vi "initialize.vi"(0 "HGF_DSCEvent":refnum<class "HGF_DSCEvent.lvclass">, 3 "initializationData":variant, 5 "error in (no error)":errorcluster, 7 "binaryString":string, 8 "I8 Array":i8[](array[numeric]), 9 "prependSize? (T)":bool, 11 "byteOrder (0:big-endian, network order)":T1(ring)) -> (14 "dup HGF_DSCEvent":refnum<class "HGF_DSCEvent.lvclass">, 17 "found?":bool, 19 "error out":errorcluster)   [LabVIEW 2012, in "HGF_DSC.lvlib" / "HGF_DSCEvent.lvclass"]
doc: "This is a dynamic dispatch VI to be implemented by child classes to initialize their attributes.\n\n<B>Recommendation:</B> Use Variant for initialization data."
uses:
  HGF_DSCEvent.lvclass
  HGF_BaseClasses/HGF_NetworkVisitor/HGF_NetworkVisitor.lvclass
  HGF_BaseClasses/HGF_Event/HGF_Event.lvclass
  HGF_SV/HGF_SVEvent/HGF_SVEvent.lvclass
  HGF_DSCEvent.lvclass/HGF_DSCEvent.ctl
  HGF_DSCCommand/HGF_DSCCommand.lvclass
  HGF_DSCFactory/HGF_DSCFactory.lvclass
  HGF_DSCSubscriber/HGF_DSCSubscriber.lvclass
  HGF_BaseClasses/HGF_NetworkEvent/HGF_NetworkEvent.lvclass/HGF_NetworkEvent.lvclass
  HGF_BaseClasses/HGF_Factory/HGF_Factory.lvclass
  HGF_SV/Visitors/HGF_SVMonitorVisitor_register/HGF_SVMonitorVisitor_register.lvclass
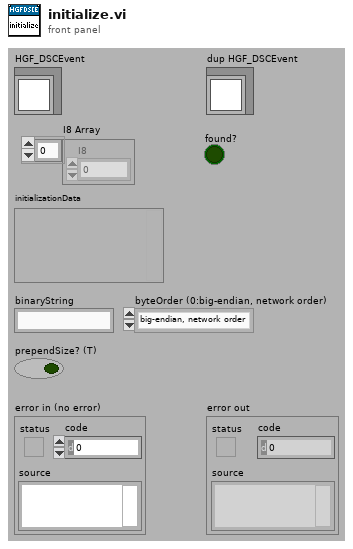
[diagram p1: front panel]
types:
  T1 = enum16{"big-endian, network order", "native, host order", "little-endian"}
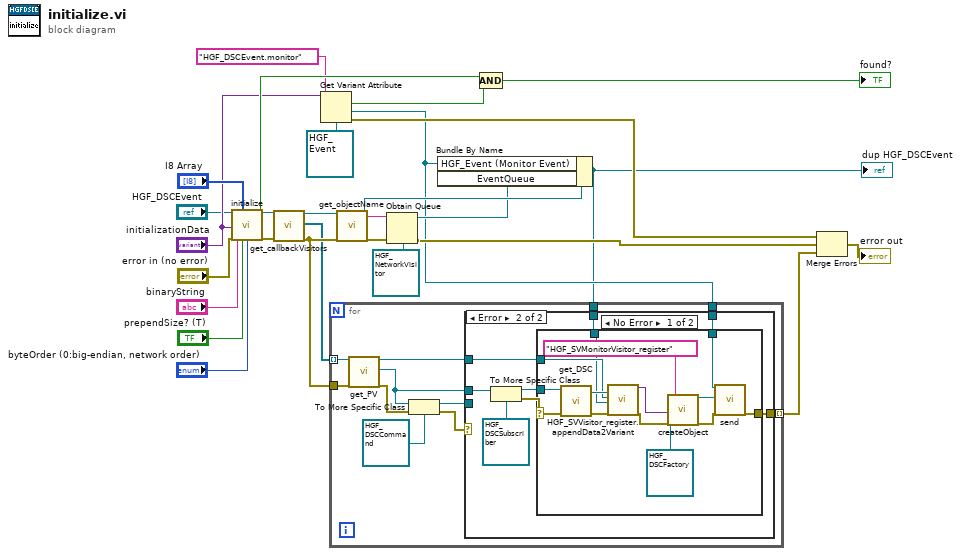
[diagram p0: block diagram]
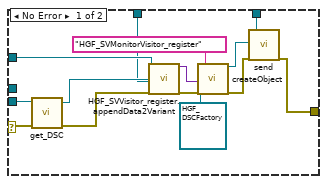
[diagram p2: hidden frame]
diagram:
  n1 = call-parent "initialize.vi"("HGF_SVEvent"="HGF_DSCEvent", "initializationData"="initializationData", "error in (no error)"="error in (no error)", "binaryString"="binaryString", "I8 Array"="I8 Array", "prependSize? (T)"="prependSize? (T)", "byteOrder (0:big-endian, network order)"="byteOrder (0:big-endian, network order)") -> ("dup HGF_SVEvent"=w6:refnum<class "HGF_DSCEvent.lvclass">, "found?"=w22:bool, "error out"=w4:errorcluster)  [unwired: 10 out]
  n2 = call "get_callbackVisitors.vi"("HGF_NetworkEvent"=w6, "error in (no error)"=w4) -> ("dup HGF_NetworkEvent"=w17:refnum<class "HGF_DSCEvent.lvclass">, "callbackVisitors"=w27:refnum<class "HGF_NetworkVisitor.lvclass">[], "error out"=w28:errorcluster)  [unwired: 15 out]
  n3 = Get Variant Attribute(Variant="initializationData", name="HGF_DSCEvent.monitor", default value (empty Variant)=refnum<class "HGF_Event.lvclass"> refnum ("HGF_BaseClasses.lvlib:HGF_Event.lvclass")) -> (found=w9:bool, value=w2:refnum<class "HGF_Event.lvclass">, error out=w5:errorcluster)  [unwired: 1 in, 1 out]
  n4 = call "get_objectName.vi"("HGF_Factory"=w17, "error in (no error)"=w28) -> ("dup HGF_Factory"=w16:refnum<class "HGF_DSCEvent.lvclass">, "objectName"=w13:string, "error out"=w15:errorcluster)  [unwired: 15 out]
  n5 = Obtain Queue(name (unnamed)=w13, element data type=refnum<class "HGF_NetworkVisitor.lvclass"> refnum ("HGF_BaseClasses.lvlib:HGF_NetworkVisitor.lvclass"), error in (no error)=w15) -> (queue out=w8:refnum<queue>, error out=w14:errorcluster)  [unwired: 2 in, 1 out]
  n6 = Bundle By Name(cluster=w16, "HGF_Event (Monitor Event)"=w2, "EventQueue"=w8) -> (w1:refnum<class "HGF_DSCEvent.lvclass">)
  "dup HGF_DSCEvent" <- w1
  n7 = for {
    tunnel: w27 -> [w39] mode=indexing
    tunnel: [w35] -> w26 mode=indexing
    tunnel: w28 -> [w31]
    tunnel: w2 -> [w30]
    tunnel: w1 -> [w29]
    n8 = call "get_PV.vi"("HGF_NetworkData"=w39, "error in (no error)"=w31) -> ("dup HGF_NetworkData"=w36:refnum<class "HGF_NetworkVisitor.lvclass">, "HGV_PVBase"=w32:refnum<class "HGF_PVBase.lvclass">, "error out"=w33:errorcluster)  [unwired: 15 out]
    n9 = To More Specific Class(target class=refnum<class "HGF_DSCCommand.lvclass"> refnum ("DSC.lvlib:HGF_DSCCommand.lvclass"), reference=w32, error in=w33) -> (specific class reference=w37:refnum<class "HGF_DSCCommand.lvclass">, error out=w38:errorcluster)
    n10 = case shown="Error" w38 {
      selector: w38 -> [w52 _]
      tunnel: w37 -> [w53 _]
      tunnel: w36 -> [w49 w59]
      tunnel: [w42 w58] -> w35
      tunnel: w32 -> [_ w56]
      tunnel: w30 -> [w50 w55]
      tunnel: w29 -> [w40 w54]
      frame No Error {
        n11 = call-dynamic "get_DSC.vi"("error in (no error)"=w52, "HGF_DSCCommand.lvclass in"=w53) -> ("error out"=w48:errorcluster, "SV"=w51:refnum<k21>)  [unwired: 8 out]
        n12 = call "HGF_SVVisitor_register.appendData2Variant.vi"("Shared Variable Control (DSC)"=w51, "HGF_NetworkVisitor"=w49, "HGF_TriggeredEvent"=w40, "error in"=w48) -> ("dup variant"=w46:variant, "error out"=w45:errorcluster)  [unwired: 14 in]
        n13 = call "createObject.vi"("HGF_Factory"=refnum<class "HGF_DSCFactory.lvclass"> refnum ("DSC.lvlib:HGF_DSCFactory.lvclass"), "initializationData"=w46, "error in (no error)"=w45, "className"="HGF_SVMonitorVisitor_register") -> ("HGF_Object"=w44:refnum<class "HGF_Factory.lvclass">, "error out"=w43:errorcluster)  [unwired: 13 in, 1 out]
        n14 = call-dynamic "send.vi"("HGF_Event"=w50, "Object"=w44, "error in (no error)"=w43) -> ("error out"=w42:errorcluster)  [unwired: 14 in, 2 out]
      }
      frame Error {
        n15 = To More Specific Class(target class=refnum<class "HGF_DSCSubscriber.lvclass"> refnum ("DSC.lvlib:HGF_DSCSubscriber.lvclass"), reference=w56) -> (specific class reference=w60:refnum<class "HGF_DSCSubscriber.lvclass">, error out=w61:errorcluster)  [unwired: 1 in]
        n16 = case shown="No Error" w61 {
          selector: w61 -> [w74 w76]
          tunnel: w60 -> [w75 _]
          tunnel: w59 -> [w72 _]
          tunnel: [w64 w76] -> w58
          tunnel: w55 -> [w63 _]
          tunnel: w54 -> [w62 _]
          frame No Error {
            n17 = call "get_DSC.vi"("error in (no error)"=w74, "HGF_DSCSubscriber.lvclass in"=w75) -> ("error out"=w71:errorcluster, "Shared Variable"=w73:refnum<k21>)  [unwired: 8 out]
            n18 = call "HGF_SVVisitor_register.appendData2Variant.vi"("Shared Variable Control (DSC)"=w73, "HGF_NetworkVisitor"=w72, "HGF_TriggeredEvent"=w62, "error in"=w71) -> ("dup variant"=w66:variant, "error out"=w65:errorcluster)  [unwired: 14 in]
            n19 = call "createObject.vi"("HGF_Factory"=refnum<class "HGF_DSCFactory.lvclass"> refnum ("DSC.lvlib:HGF_DSCFactory.lvclass"), "initializationData"=w66, "error in (no error)"=w65, "className"="HGF_SVMonitorVisitor_register") -> ("HGF_Object"=w70:refnum<class "HGF_Factory.lvclass">, "error out"=w69:errorcluster)  [unwired: 13 in, 1 out]
            n20 = call-dynamic "send.vi"("HGF_Event"=w63, "Object"=w70, "error in (no error)"=w69) -> ("error out"=w64:errorcluster)  [unwired: 14 in, 2 out]
          }
          frame Error {
          }
        }
      }
    }
  }
  n21 = Compound Arithmetic op=AND(w22, w9) -> (→"found?":bool)
  n22 = Merge Errors(w5, w14, w26) -> (→"error out":errorcluster)
